vi "CurveTrace_Single_Meas.vi"(5 "offset":dbl format="%#_13g", 7 "Base Gate Bias Value":dbl format="%#_13g", 11 "Test Params Cluster":T1={"Test Freq. (Hz)"=1702.3933752476319, "Output Signal Amplitude\nVolts Pk"=0.1, "Sampling Time (s)"=0.01, "Sampling Rate (Hz)"=250000.0, "Output Channel"="Dev3/ao0", "Current Channel"="Dev3/ai1", "Voltage Channel"="Dev3/ai0", "Trigger Channel"="/Dev3/ao/StartTrigger", "Number of runs"=5, "BaseGateBias Channel"="Dev3/ao0"}) -> (0 "Current Complex":cdb=0.1092230559688666-0.017870132117080606i, 1 "Voltage Complex":cdb=-0.17452167799153867-1.07754869267134i, 2 "Time domain Current":waveform(dbl)(graph)={"t0"=timestamp(3724535126.9386544 s since 1904-01-01), "dt"=3.999999999999989e-06, "Y"=array[2500 elements], "attributes"=variant("NI_ChannelName"=variant(string "Dev3/ai1"), "NI_UnitDescription"=variant(string "Volts"))}, 3 "Time domain Voltage":waveform(dbl)(graph)={"t0"=timestamp(3724535127.000671 s since 1904-01-01), "dt"=3.999999999999989e-06, "Y"=array[2500 elements], "attributes"=variant("NI_ChannelName"=variant(string "Dev3/ai0"), "NI_UnitDescription"=variant(string "Volts"))})   [LabVIEW 2022 SP3]
uses:
  <vilib>/DAQmx/write.llb/DAQmx Write (Analog DBL 1Chan 1Samp).vi
  <vilib>/DAQmx/write.llb/DAQmx Write (Analog Wfm 1Chan NSamp).vi
  <vilib>/DAQmx/read.llb/DAQmx Read (Analog 1D Wfm NChan NSamp).vi
  <vilib>/DAQmx/create/channels.llb/DAQmx Create Channel (AO-Voltage-Basic).vi
  <vilib>/DAQmx/miscellaneous.llb/DAQmx Fill In Error Info.vi
  <vilib>/DAQmx/create/channels.llb/DAQmx Create Channel (AI-Voltage-Basic).vi
  <vilib>/DAQmx/configure/timing.llb/DAQmx Timing (Sample Clock).vi
  <vilib>/DAQmx/configure/trigger.llb/DAQmx Start Trigger (Digital Edge).vi
  <vilib>/measure/matone.llb/Extract Single Tone Information 1 Chan.vi
  <vilib>/measure/NI_MABase.lvlib
  <vilib>/measure/NI_MAPro.lvlib
panel:
  in  "phase":dbl format="%.2p"
  out "Waveform Graph":waveform(dbl)(graph)
  out "Test Freq. (Hz)":dbl=1702.3933752476319
  out "Mag Current":dbl=0.1106752798824565
  in  "Use LabView\nSignal Detect":bool=TRUE
  out "detected phase (Rad)":dbl=4.551821517545998
  out "detected amplitude":dbl=1.0915901250774929 format="%.2p"
  in  "search (+/- % of Fsampl.)":dbl
  in  "advanced search":T2={"approx freq. (optional)"=-1.0, "search (+/- % of Fsampl.)"=5.0} {"search (+/- % of Fsampl.)" format="%0.2p"; "approx freq. (optional)" format="%0.2p"}
  out "Detected Time domain Current 2":waveform(dbl)(graph)={"t0"=timestamp(2.12 s since 1904-01-01), "dt"=4e-06, "Y"=array[2500 elements]}
  out "Detected Time domain Voltage 2":waveform(dbl)(graph)={"t0"=timestamp(2.13 s since 1904-01-01), "dt"=4e-06, "Y"=array[2500 elements]}
  out "detected frequency 2":dbl=1700.0000000000045 format="%.2p"
  out "detected frequency":dbl=1700.0000000000045 format="%.2p"
  out "Current phase (deg)":dbl=-0.16217447631966198 format="%.2p"
  out "Voltage phase (deg)":dbl=260.8001620522193 format="%.2p"
  in  "CurentRangeMax":dbl=5.0 format="%0.2f"
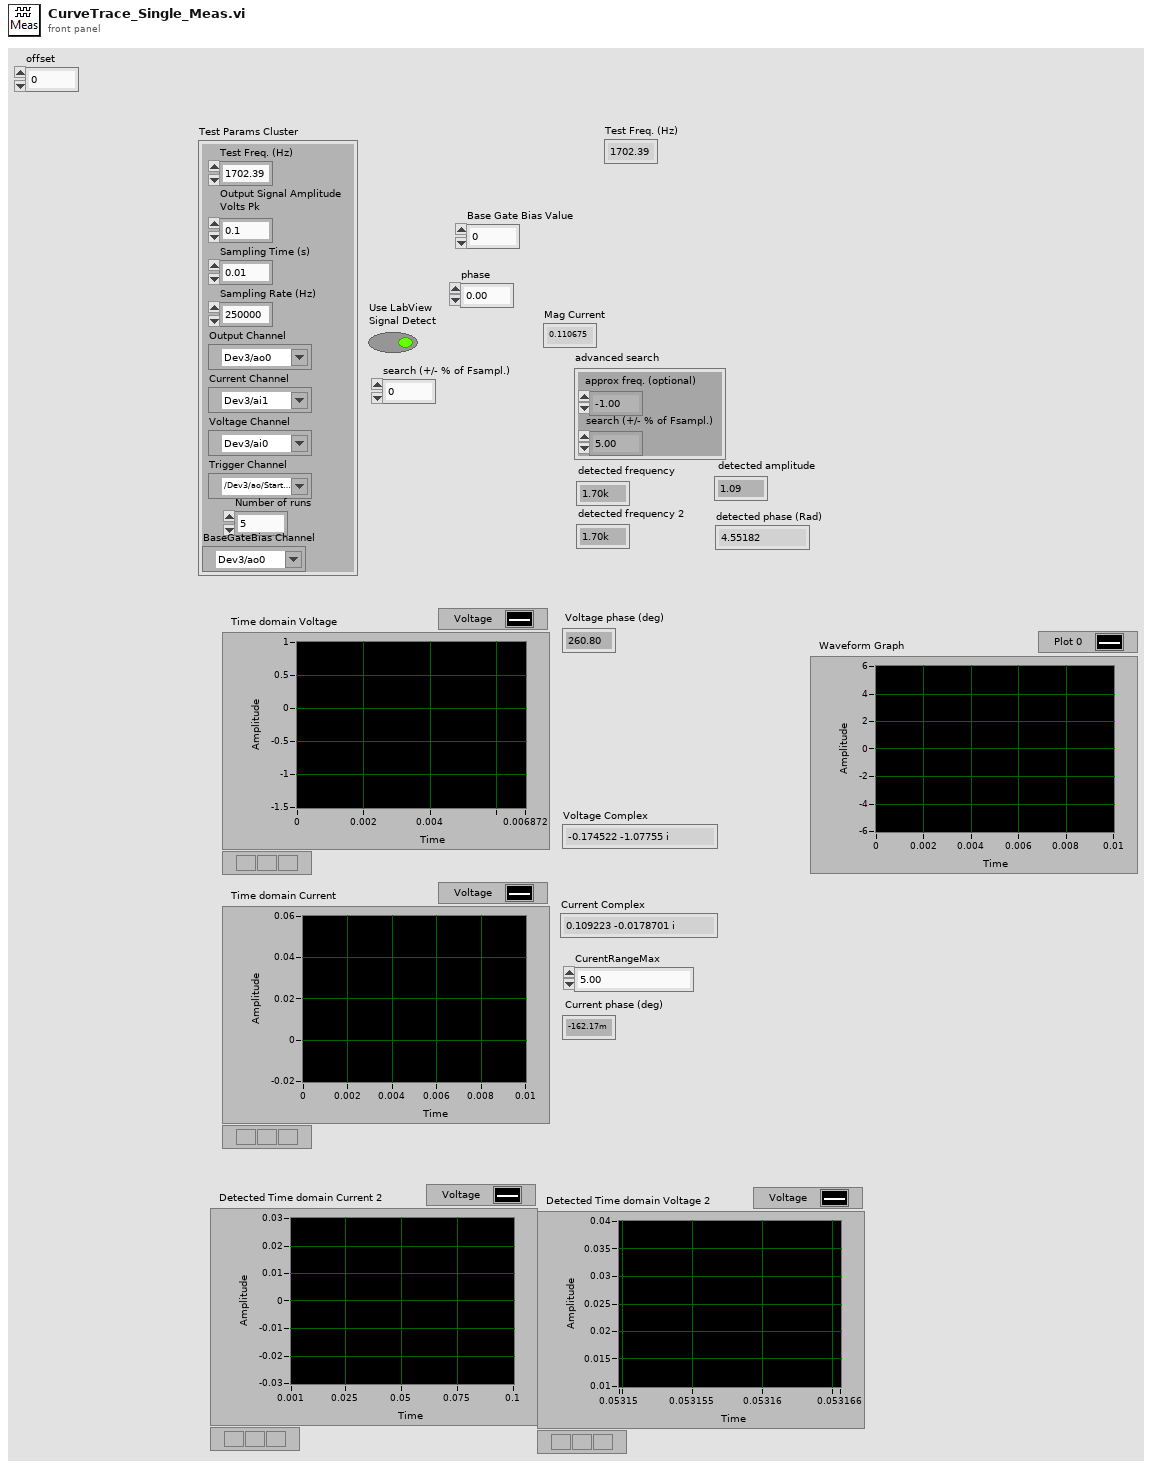
[diagram p1: front panel]
types:
  T1 = cluster{"Test Freq. (Hz)":dbl, "Output Signal Amplitude\nVolts Pk":dbl, "Sampling Time (s)":dbl, "Sampling Rate (Hz)":dbl, "Output Channel":tag, "Current Channel":tag, "Voltage Channel":tag, "Trigger Channel":tag, "Number of runs":i32, "BaseGateBias Channel":tag}
  T2 = cluster{"approx freq. (optional)":dbl, "search (+/- % of Fsampl.)":dbl}
  T3 = enum32{"none", "input signal", "detected signal", "residual signal"}
  T4 = cluster{"exported time signal":waveform(dbl), "exported spectrum (dB)":cluster{"f0":dbl, "df":dbl, "dB Spectrum (Hann)":dbl[]}}
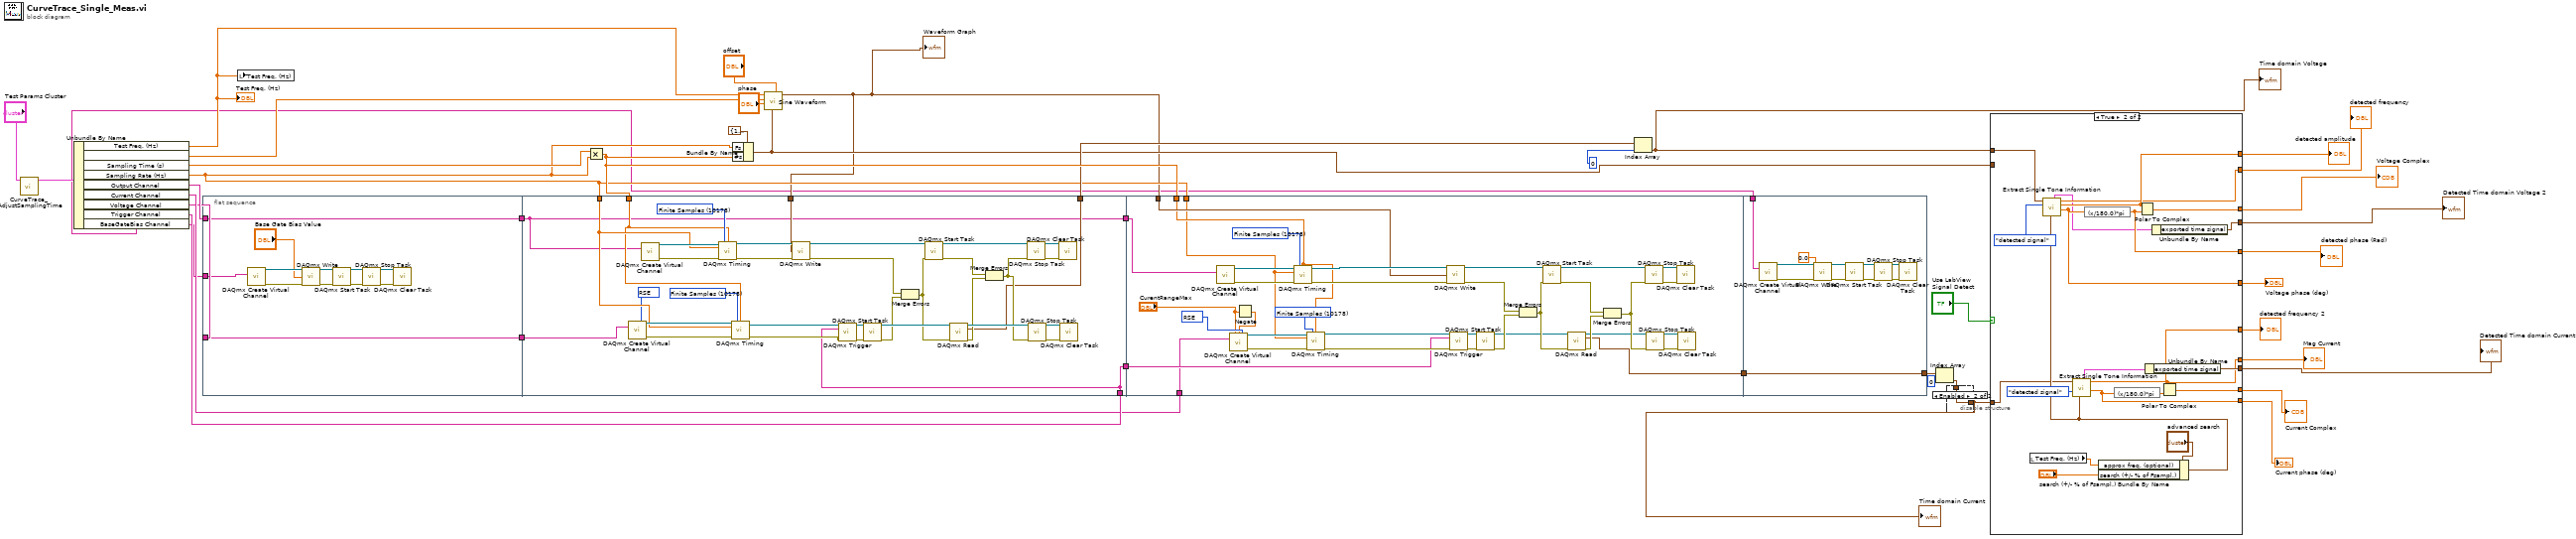
[diagram p0: block diagram]
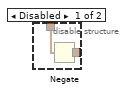
[diagram p2: hidden frame]
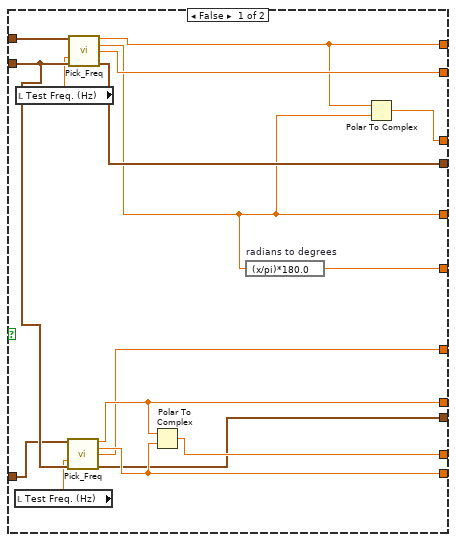
[diagram p3: hidden frame]
diagram:
  n1 = call "CurveTrace_AdjustSamplingTime.vi"("Test Params Cluster"="Test Params Cluster") -> ("output cluster"=w8:T1)  [unwired: 10 in]
  n2 = Unbundle By Name(w8) -> ("Test Freq. (Hz)"=w16:dbl, "Output Signal Amplitude\nVolts Pk"=w15:dbl, "Sampling Time (s)"=w14:dbl, "Sampling Rate (Hz)"=w13:dbl, "Output Channel"=w11:tag, "Current Channel"=w10:tag, "Voltage Channel"=w9:tag, "Trigger Channel"=w12:tag, "BaseGateBias Channel"=w1:tag)
  "Test Freq. (Hz)" <- w16
  n3 = flat-sequence {
    tunnel: w9 -> [w52]
    tunnel: w11 -> [w53]
    tunnel: [w53] -> w7
    tunnel: [w52] -> w6
    tunnel: w1 -> [w51]
    tunnel: w13 -> [w65]
    tunnel: w38 -> [w64]
    tunnel: w4 -> [w62]
    tunnel: [w57] -> w35
    tunnel: [w56] -> w39
    tunnel: [w54] -> w28
    tunnel: w12 -> [w54]
    tunnel: w7 -> [w56]
    tunnel: w6 -> [w55]
    tunnel: w39 -> [w96]
    tunnel: w4 -> [w94]
    tunnel: w38 -> [w93]
    tunnel: w13 -> [w92]
    tunnel: w28 -> [w89]
    tunnel: w10 -> [w88]
    tunnel: [w95] -> w2
    tunnel: [w134] -> w32
    tunnel: w2 -> [w134]
    tunnel: w1 -> [w124]
    frame #0 {
      n4 = call-poly <vilib>:"DAQmx Create Virtual Channel.vi"("physical channels"=w51) -> ("task out"=w50:refnum<k21>, "error out"=w43:errorcluster)  [unwired: 13 in]
      n5 = call-poly <vilib>:"DAQmx Write.vi"("task/channels in"=w50, "data"="Base Gate Bias Value", "error in"=w43) -> ("task out"=w49:refnum<k21>, "error out"=w44:errorcluster)  [unwired: 10 in, 1 out]
      n6 = call <vilib>:"DAQmx Start Task.vi"("task/channels in"=w49, "error in"=w44) -> ("task out"=w48:refnum<k21>, "error out"=w45:errorcluster)  [unwired: 12 in]
      n7 = call <vilib>:"DAQmx Stop Task.vi"("task/channels in"=w48, "error in"=w45) -> ("task out"=w47:refnum<k21>, "error out"=w46:errorcluster)  [unwired: 12 in]
      n8 = call <vilib>:"DAQmx Clear Task.vi"("task in"=w47, "error in"=w46) -> ()  [unwired: 13 in, 1 out]
    }
    frame #1 {
      w63 = 10083 items=["Default"=-1, "RSE"=10083, "NRSE"=10078, "Differential"=10106, "Pseudodifferential"=12529] ("input terminal configuration")
      w77 = 10178 items=["Finite Samples"=10178, "Continuous Samples"=10123, "Hardware Timed Single Point"=12522] ("sample mode")
      w80 = 10178 items=["Finite Samples"=10178, "Continuous Samples"=10123, "Hardware Timed Single Point"=12522] ("sample mode")
      n9 = call-poly <vilib>:"DAQmx Create Virtual Channel.vi"("input terminal configuration"=w63, "physical channels"=w55) -> ("task out"=w78:refnum<k21>, "error out"=w79:errorcluster)  [unwired: 12 in]
      n10 = call-poly <vilib>:"DAQmx Create Virtual Channel.vi"("physical channels"=w56) -> ("task out"=w87:refnum<k21>, "error out"=w83:errorcluster)  [unwired: 13 in]
      n11 = call-poly <vilib>:"DAQmx Timing.vi"("task/channels in"=w87, "sample mode"=w80, "samples per channel"=w64, "rate"=w65, "error in"=w83) -> ("task out"=w86:refnum<k21>, "error out"=w84:errorcluster)  [unwired: 9 in]
      n12 = call-poly <vilib>:"DAQmx Timing.vi"("task/channels in"=w78, "sample mode"=w77, "samples per channel"=w64, "rate"=w65, "error in"=w79) -> ("task out"=w76:refnum<k21>, "error out"=w75:errorcluster)  [unwired: 9 in]
      n13 = call-poly <vilib>:"DAQmx Write.vi"("task/channels in"=w86, "data"=w62, "error in"=w84) -> ("task out"=w85:refnum<k21>, "error out"=w67:errorcluster)  [unwired: 10 in, 1 out]
      n14 = call-poly <vilib>:"DAQmx Trigger.vi"("task/channels in"=w76, "source"=w54, "error in"=w75) -> ("task out"=w73:refnum<k21>, "error out"=w74:errorcluster)  [unwired: 11 in]
      n15 = call <vilib>:"DAQmx Start Task.vi"("task/channels in"=w73, "error in"=w74) -> ("task out"=w72:refnum<k21>, "error out"=w68:errorcluster)  [unwired: 12 in]
      n16 = Merge Errors(w67, w68) -> (w66:errorcluster)
      n17 = call <vilib>:"DAQmx Start Task.vi"("task/channels in"=w85, "error in"=w66) -> ("task out"=w82:refnum<k21>, "error out"=w59:errorcluster)  [unwired: 12 in]
      n18 = call-poly <vilib>:"DAQmx Read.vi"("task/channels in"=w72, "error in"=w66) -> ("task out"=w69:refnum<k21>, "data"=w57:waveform(dbl)[], "error out"=w60:errorcluster)  [unwired: 11 in]
      n19 = Merge Errors(w59, w60) -> (w58:errorcluster)
      n20 = call <vilib>:"DAQmx Stop Task.vi"("task/channels in"=w82, "error in"=w58) -> ("task out"=w81:refnum<k21>, "error out"=w61:errorcluster)  [unwired: 12 in]
      n21 = call <vilib>:"DAQmx Stop Task.vi"("task/channels in"=w69, "error in"=w58) -> ("task out"=w70:refnum<k21>, "error out"=w71:errorcluster)  [unwired: 12 in]
      n22 = call <vilib>:"DAQmx Clear Task.vi"("task in"=w81, "error in"=w61) -> ()  [unwired: 13 in, 1 out]
      n23 = call <vilib>:"DAQmx Clear Task.vi"("task in"=w70, "error in"=w71) -> ()  [unwired: 13 in, 1 out]
    }
    frame #2 {
      w119 = 10083 items=["Default"=-1, "RSE"=10083, "NRSE"=10078, "Differential"=10106, "Pseudodifferential"=12529] ("input terminal configuration")
      w107 = 10178 items=["Finite Samples"=10178, "Continuous Samples"=10123, "Hardware Timed Single Point"=12522] ("sample mode")
      w104 = 10178 items=["Finite Samples"=10178, "Continuous Samples"=10123, "Hardware Timed Single Point"=12522] ("sample mode")
      n24 = call-poly <vilib>:"DAQmx Create Virtual Channel.vi"("physical channels"=w96) -> ("task out"=w97:refnum<k21>, "error out"=w101:errorcluster)  [unwired: 13 in]
      n25 = Negate(x="CurentRangeMax") -> (-x=w90:dbl)
      n26 = call-poly <vilib>:"DAQmx Create Virtual Channel.vi"("maximum value"="CurentRangeMax", "minimum value"=w90, "input terminal configuration"=w119, "physical channels"=w88) -> ("task out"=w106:refnum<k21>, "error out"=w105:errorcluster)  [unwired: 10 in]
      n27 = call-poly <vilib>:"DAQmx Timing.vi"("task/channels in"=w97, "sample mode"=w104, "samples per channel"=w93, "rate"=w92, "error in"=w101) -> ("task out"=w98:refnum<k21>, "error out"=w100:errorcluster)  [unwired: 9 in]
      n28 = call-poly <vilib>:"DAQmx Timing.vi"("task/channels in"=w106, "sample mode"=w107, "samples per channel"=w93, "rate"=w92, "error in"=w105) -> ("task out"=w108:refnum<k21>, "error out"=w109:errorcluster)  [unwired: 9 in]
      n29 = call-poly <vilib>:"DAQmx Write.vi"("task/channels in"=w98, "data"=w94, "error in"=w100) -> ("task out"=w99:refnum<k21>, "error out"=w117:errorcluster)  [unwired: 10 in, 1 out]
      n30 = call-poly <vilib>:"DAQmx Trigger.vi"("task/channels in"=w108, "source"=w89, "error in"=w109) -> ("task out"=w111:refnum<k21>, "error out"=w110:errorcluster)  [unwired: 11 in]
      n31 = call <vilib>:"DAQmx Start Task.vi"("task/channels in"=w111, "error in"=w110) -> ("task out"=w112:refnum<k21>, "error out"=w116:errorcluster)  [unwired: 12 in]
      n32 = Merge Errors(w117, w116) -> (w118:errorcluster)
      n33 = call <vilib>:"DAQmx Start Task.vi"("task/channels in"=w99, "error in"=w118) -> ("task out"=w102:refnum<k21>, "error out"=w122:errorcluster)  [unwired: 12 in]
      n34 = call-poly <vilib>:"DAQmx Read.vi"("task/channels in"=w112, "error in"=w118) -> ("task out"=w115:refnum<k21>, "data"=w95:waveform(dbl)[], "error out"=w121:errorcluster)  [unwired: 11 in]
      n35 = Merge Errors(w122, w121) -> (w123:errorcluster)
      n36 = call <vilib>:"DAQmx Stop Task.vi"("task/channels in"=w102, "error in"=w123) -> ("task out"=w103:refnum<k21>, "error out"=w120:errorcluster)  [unwired: 12 in]
      n37 = call <vilib>:"DAQmx Stop Task.vi"("task/channels in"=w115, "error in"=w123) -> ("task out"=w114:refnum<k21>, "error out"=w113:errorcluster)  [unwired: 12 in]
      n38 = call <vilib>:"DAQmx Clear Task.vi"("task in"=w103, "error in"=w120) -> ()  [unwired: 13 in, 1 out]
      n39 = call <vilib>:"DAQmx Clear Task.vi"("task in"=w114, "error in"=w113) -> ()  [unwired: 13 in, 1 out]
    }
    frame #3 {
      n40 = call-poly <vilib>:"DAQmx Create Virtual Channel.vi"("physical channels"=w124) -> ("task out"=w133:refnum<k21>, "error out"=w126:errorcluster)  [unwired: 13 in]
      n41 = call-poly <vilib>:"DAQmx Write.vi"("task/channels in"=w133, "data"=0.0, "error in"=w126) -> ("task out"=w132:refnum<k21>, "error out"=w127:errorcluster)  [unwired: 10 in, 1 out]
      n42 = call <vilib>:"DAQmx Start Task.vi"("task/channels in"=w132, "error in"=w127) -> ("task out"=w131:refnum<k21>, "error out"=w128:errorcluster)  [unwired: 12 in]
      n43 = call <vilib>:"DAQmx Stop Task.vi"("task/channels in"=w131, "error in"=w128) -> ("task out"=w130:refnum<k21>, "error out"=w129:errorcluster)  [unwired: 12 in]
      n44 = call <vilib>:"DAQmx Clear Task.vi"("task in"=w130, "error in"=w129) -> ()  [unwired: 13 in, 1 out]
    }
  }
  n45 = local write "Test Freq. (Hz)"(w16) -> ()
  n46 = Multiply(x=w14, y=w13) -> (x*y=w38:dbl)
  n47 = Bundle By Name(cluster=cluster{"Fs":dbl, "#s":dbl} {"Fs"=1000.0, "#s"=1000.0} ("sampling info"), "Fs"=w13, "#s"=w38) -> (w18:cluster{"Fs":dbl, "#s":dbl})
  n48 = call <vilib>:"Sine Waveform.vi"("offset"="offset", "sampling info"=w18, "phase"="phase", "amplitude"=w15, "frequency"=w16) -> ("signal out"=w4:waveform(dbl))  [unwired: 5 in, 1 out]
  "Waveform Graph" <- w4
  n49 = Index Array(array=w35, index=0) -> (element=w27:waveform(dbl))
  "Time domain Voltage" <- w27
  n50 = Index Array(array=w32, index=0) -> (element=w30:waveform(dbl))
  n51 = disable-structure shown="Enabled" {
    disable-tunnel: w30 -> [w136 w137]
    disable-tunnel: [w135 w137] -> w17
    frame Disabled {
      n52 = Negate(x=w136) -> (-x=w135:waveform(dbl))
    }
    frame Enabled {
    }
  }
  "Time domain Current" <- w17
  n53 = case shown="True" "Use LabView\nSignal Detect" {
    tunnel: [w143 w175] -> w37
    tunnel: [w142 w174] -> w36
    tunnel: [w144 w172] -> w31
    tunnel: [w152 w171] -> w29
    tunnel: w27 -> [w153 w165]
    tunnel: [w146 w164] -> w25
    tunnel: [w149 w163] -> w24
    tunnel: [w150 w162] -> w23
    tunnel: [w145 w161] -> w22
    tunnel: [w151 w156] -> w21
    tunnel: [w147 w158] -> w20
    tunnel: [w148 w157] -> w19
    tunnel: w18 -> [w141 _]
    tunnel: w17 -> [w140 w155]
    frame False {
      n54 = local read "Test Freq. (Hz)"() -> (w139:dbl)
      n55 = local read "Test Freq. (Hz)"() -> (w138:dbl)
      n56 = call "Pick_Freq.vi"("time signal"=w140, "RX frequency"=w139, "sampling info"=w141) -> ("Mag"=w151:dbl, "Phase"=w150:dbl, "actual freq"=w146:dbl, "signal out"=w147:waveform(dbl))  [unwired: 9 in]
      n57 = call "Pick_Freq.vi"("time signal"=w153, "RX frequency"=w138, "sampling info"=w141) -> ("Mag"=w143:dbl, "Phase"=w142:dbl, "actual freq"=w152:dbl, "signal out"=w148:waveform(dbl))  [unwired: 9 in]
      n58 = Polar To Complex(1:w150, 2:w151) -> (0:w149:cdb)
      n59 = expression code="(x/pi)*180.0" "radians to degrees"(w142) -> (w145:dbl)
      n60 = Polar To Complex(1:w142, 2:w143) -> (0:w144:cdb)
    }
    frame True {
      n61 = local read "Test Freq. (Hz)"() -> (w154:dbl)
      n62 = Bundle By Name(cluster="advanced search", "approx freq. (optional)"=w154, "search (+/- % of Fsampl.)"="search (+/- % of Fsampl.)") -> (w167:T2)
      n63 = call-poly <vilib>:"Extract Single Tone Information.vi"("advanced search"=w167, "export mode"=T3."detected signal", "time signal in"=w165) -> ("detected phase (deg)"=w161:dbl, "detected amplitude"=w175:dbl, "detected frequency"=w171:dbl, "exported signals"=w160:T4)  [unwired: 3 in, 2 out]
      n64 = call-poly <vilib>:"Extract Single Tone Information.vi"("advanced search"=w167, "export mode"=T3."detected signal", "time signal in"=w155) -> ("detected phase (deg)"=w162:dbl, "detected amplitude"=w156:dbl, "detected frequency"=w164:dbl, "exported signals"=w159:T4)  [unwired: 3 in, 2 out]
      n65 = expression code="(x/180.0)*pi" ("degrees to radians")(w161) -> (w174:dbl)
      n66 = expression code="(x/180.0)*pi" ("degrees to radians")(w162) -> (w173:dbl)
      n67 = Polar To Complex(1:w174, 2:w175) -> (0:w172:cdb)
      n68 = Unbundle By Name(w159) -> ("exported time signal"=w158:waveform(dbl))
      n69 = Unbundle By Name(w160) -> ("exported time signal"=w157:waveform(dbl))
      n70 = Polar To Complex(1:w173, 2:w156) -> (0:w163:cdb)
    }
  }
  "Voltage Complex" <- w31
  "detected frequency" <- w29
  "Detected Time domain Voltage 2" <- w19
  "Detected Time domain Current 2" <- w20
  "detected amplitude" <- w37
  "detected phase (Rad)" <- w36
  "detected frequency 2" <- w25
  "Current Complex" <- w24
  "Current phase (deg)" <- w23
  "Voltage phase (deg)" <- w22
  "Mag Current" <- w21
